vi "Average.vi"() -> ()   [LabVIEW 2011, in "Diamond Universal Driver.lvlib"]
uses:
  Diamond Universal Driver.lvlib
  Controls/dscBool.ctl
  Controls/board type.ctl
  Controls/dsccb.ctl
  constants.vi
  Controls/gain.ctl
  Controls/dscADSettings.ctl
  Controls/dscADScan.ctl
  support/dlls/mm32at.dll
  Controls/dscAIOint.ctl
  IO/DSCS.ctl
panel:
  out "status":T1 {"analog" items=["FALSE", "TRUE"]}
  out "aioint":T3 {"ch_align" items=["FALSE", "TRUE"]; "fifo en" items=["FALSE", "TRUE"]; "int clk gate" items=["FALSE", "TRUE"]; "ext gate en" items=["FALSE", "TRUE"]; "intclk" items=["FALSE", "TRUE"]; "cycle" items=["FALSE", "TRUE"]}
  out "ctVal":i32
  out "error out 2":errorcluster
  out "error":u8
  out "current time":timestamp
  out "sample_val":dbl[](array[numeric])
  out "error out":errorcluster
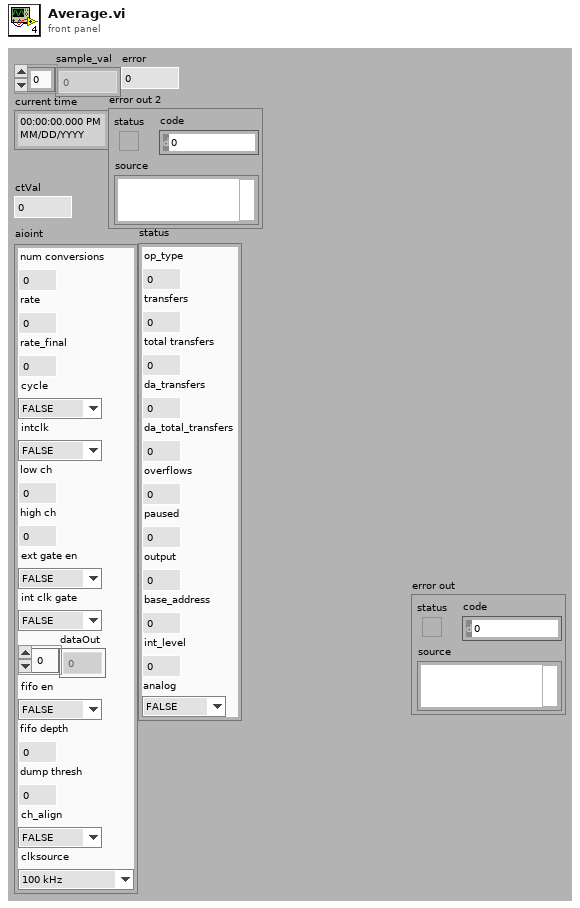
[diagram p1: front panel]
types:
  T1 = typedef "Diamond Universal Driver.lvlib/DSCS.ctl" = cluster{"op_type":u8, "transfers":u32, "total transfers":u32, "da_transfers":u32, "da_total_transfers":u32, "overflows":u32, "paused":u8, "output":u8, "base_address":u16, "int_level":u8, "analog":T2}
  T2 = typedef "dscBool.ctl" = i32
  T3 = typedef "Diamond Universal Driver.lvlib/dscAIOint.ctl" = cluster{"num conversions":u32, "rate":sgl, "rate_final":sgl, "cycle":T2, "intclk":T2, "low ch":u8, "high ch":u8, "ext gate en":T2, "int clk gate":T2, "dataOut":i16[], "fifo en":T2, "fifo depth":u16, "dump thresh":u32, "ch_align":T2, "clksource":enum8{"100 kHz", "1 MHz"}}
  T4 = typedef "dscADSettings.ctl" = cluster{"current_ch":u8, "gain":T5, "range":enum8{"RANGE_5", "RANGE_10"}, "polarity":enum16{"BIPOLAR", "UNIPOLAR"}, "load cal":u8, "scan_int":enum8{"20", "15", "10", "5", "9", "4"}, "addiff":enum8{"Single Ended", "Differential"}}
  T5 = typedef "gain.ctl" = enum8{"GAIN_1", "GAIN_2", "GAIN_8"}
  T6 = typedef "board type.ctl" = u8
  T7 = typedef "dsccb.ctl" = cluster{"board type":T6, "board num":i16, "base addr":u16, "int level":u8, "RMM external trig":T2, "RMM external trig c3":T2, "EMM IOAdd":u16[], "EMM IOInterrupt":u16[], "clkfreq0":enum8{"10 MHz", "1 MHz"}, "clkfreq1":enum8{"10 MHz", "1 MHz"}, "clksel1":enum8{"Internal (clkfrq1)", "External"}, "address space":dbl, "DAC cfg":u8, "clck_freq":i32, "dma_level":u8, "int_lvl 1":u8, "int_lvl 2":u8, "int_lvl 3":u8, "fpga":u16, "smm_ad_res":u8, "RMM mode 16bit":T2, "RMM DAC 0_3 ext en":T2, "RMM DAC 4_7 ext en":T2}
  T8 = typedef "dscADScan.ctl" = cluster{"low channel":u8, "high channel":u8, "sample_val":u16[], "gain":T5}
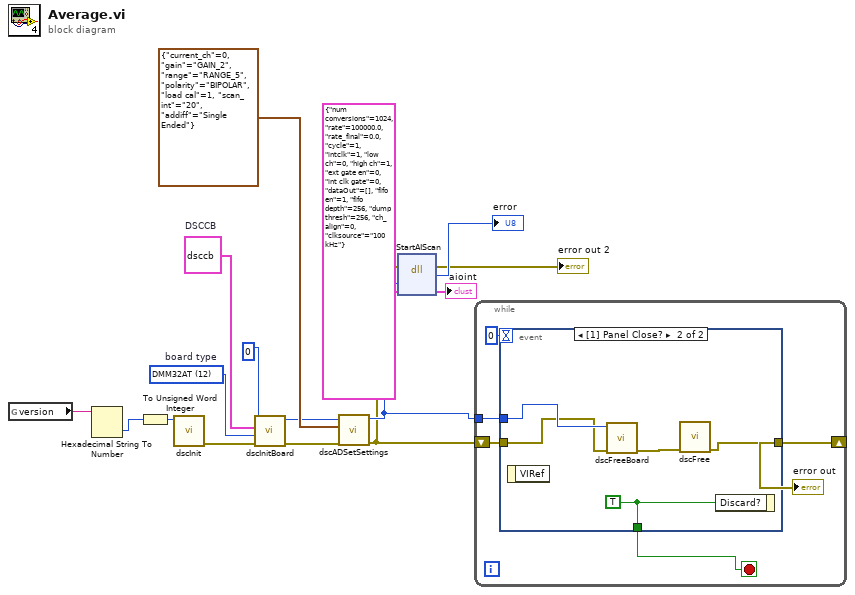
[diagram p0: block diagram]
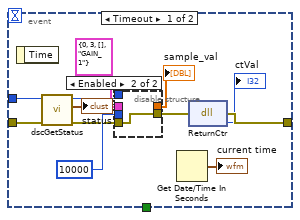
[diagram p2: hidden frame]
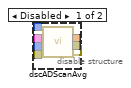
[diagram p3: hidden frame]
diagram:
  w12 = T6 12 items=["DMM16"=0, "RMM"=1, "TMM"=2, "OPMM"=3, "DMM"=4, "SMM"=5, "GMM"=6, "QMM"=7, "ZMM"=8, "PMM"=9, "OMM"=10, "RMM416"=11, "DMM32AT"=12, "EMMDIO"=13, "RMM1612"=14, "DMMAT"=15, "DMM16AT"=16, "IR104"=17, "EMM8"=18, "PROM"=19, "HERCEBX"=20, "CPT"=21, "DMM48AT"=22, "OMMIO"=23, "DIO82C55"=24, "ATHENA"=25, "METIS"=26, "DMM32XAT"=27, "ELEKTRA"=28, "GPIO11_9513"=29, "GPIO11_DIO"=30, "GPIO21"=31, "PSD"=32, "ATHENAII"=33, "DMM32DXAT"=34, "HELIOS"=35, "NEPTUNE"=36, "TEST"=126, "RAW"=127, "DRVR"=255]  # board type
  w10 = T7 {"board type"=12, "board num"=1, "base addr"=768, "int level"=3, "RMM external trig"=0, "RMM external trig c3"=0, "EMM IOAdd"=[0, 0, 0, 0, 0, 0, 0, 0], "EMM IOInterrupt"=[0, 0, 0, 0, 0, 0, 0, 0], "clkfreq0"=enum."10 MHz", "clkfreq1"=enum."10 MHz", "clksel1"=enum."Internal (clkfrq1)", "address space"=0.0, "DAC cfg"=0, "clck_freq"=0, "dma_level"=0, "int_lvl 1"=0, "int_lvl 2"=0, "int_lvl 3"=0, "fpga"=0, "smm_ad_res"=0, "RMM mode 16bit"=0, "RMM DAC 0_3 ext en"=0, "RMM DAC 4_7 ext en"=0}  # DSCCB
  n1 = global read "constants.vi" "version"() -> (w16:string)
  n2 = Hexadecimal String To Number(string=w16) -> (number=w14:u32)  [unwired: 2 in, 1 out]
  n3 = To Unsigned Word Integer(number=w14) -> (unsigned 16bit integer=w15:u16)
  n4 = call "dscInit.vi"("versionIn"=w15) -> ("error out"=w13:errorcluster)  [unwired: 9 in, 1 out]
  n5 = call "dscInitBoard.vi"("error in"=w13, "board type"=w12, "DSCCB"=w10, 11:u16 0 ("boardHandle")) -> ("error out"=w7:errorcluster, "boardHandleOut"=w8:i16)  [unwired: 5 in, 1 out]
  n6 = call "dscADSetSettings.vi"("error in"=w7, "adSettingsIn"=T4 {"current_ch"=0, "gain"=enum."GAIN_2", "range"=enum."RANGE_5", "polarity"=enum."BIPOLAR", "load cal"=1, "scan_int"=enum."20", "addiff"=enum."Single Ended"}, "boardIn"=w8) -> ("error out"=w4:errorcluster, "boardOut"=w5:i16)  [unwired: 6 in, 1 out]
  n7 = dll-call lib="C:/Users/mrichardson/Documents/Web Based Version Control SW/Reusable/Diamond Universal Driver/support/dlls/mm32at.dll" fn="StartAIScan"(error in=w4, "board"=w5, "aioint"=T3 {"num conversions"=1024, "rate"=100000.0, "rate_final"=0.0, "cycle"=1, "intclk"=1, "low ch"=0, "high ch"=1, "ext gate en"=0, "int clk gate"=0, "dataOut"=[], "fifo en"=1, "fifo depth"=256, "dump thresh"=256, "ch_align"=0, "clksource"=enum."100 kHz"} ("dscAIOint")) -> (error out=→"error out 2":errorcluster, "error"=→"error":u8, "aioint"=→"aioint":T3)  [unwired: 3 in, 1 out]
  n8 = while {
    tunnel: w5 -> [w19]
    shift-right: [w17] -> _
    shift-left: w4 -> [w18]
    stop <- w20 stop-if-true
    n9 = event shown="[1] Panel Close?" {
      selector: _ -> [_ _]
      dyn-events: _ -> [_ _]
      timeout: 0 -> [_ _]
      tunnel: [_ w45] -> w20
      tunnel: w19 -> [w26 w42]
      tunnel: w18 -> [w25 w41]
      tunnel: [w28 w43] -> w17
      event Timeout {
        n10 = event-data() -> ()  [unwired: 1 in, 1 out]
        n11 = call "dscGetStatus.vi"("error in"=w25, "board"=w26) -> ("error out"=w23:errorcluster, "status"=→"status":T1, "boardOut"=w24:i16)  [unwired: 7 in]
        n12 = disable-structure shown="Enabled" {
          disable-tunnel: [w39 _] -> w33
          disable-tunnel: 10000 ("count") -> [w38 _]
          disable-tunnel: T8 {"low channel"=0, "high channel"=3, "sample_val"=[], "gain"=enum."GAIN_1"} ("dscadscan") -> [w37 _]
          disable-tunnel: [w36 w40] -> w29
          disable-tunnel: w24 -> [w35 _]
          disable-tunnel: w23 -> [w34 w40]
          frame Disabled {
            n13 = call "dscADScanAvg.vi"("error in"=w34, "count"=w38, "dscadscan"=w37, "board"=w35) -> ("error out"=w36:errorcluster, "DataOut"=w39:cluster{"time":timestamp, "sample_val":sgl[]})  [unwired: 5 in, 1 out]
          }
          frame Enabled {
          }
        }
        "sample_val" <- w33
        n14 = Get Date/Time In Seconds() -> (seconds since 1Jan1904=→"current time":timestamp)
        n15 = dll-call lib="C:/Users/mrichardson/Documents/Web Based Version Control SW/Reusable/Diamond Universal Driver/support/dlls/mm32at.dll" fn="ReturnCtr"(error in=w29) -> (error out=w28:errorcluster, "ctVal"=→"ctVal":i32)  [unwired: 2 in, 1 out]
      }
      event Panel Close? {
        w45 = TRUE ("Discard?")
        n16 = event-data() -> ()  [unwired: 1 in, 1 out]
        n17 = call "dscFreeBoard.vi"("error in"=w41, "boardIn"=w42) -> ("error out"=w44:errorcluster)  [unwired: 8 in, 1 out]
        n18 = call "dscFree.vi"("error in"=w44) -> ("error out"=w43:errorcluster)  [unwired: 10 in]
        n19 = event-data("Discard?"=w45) -> ()  [unwired: 1 in, 1 out]
      }
    }
    "error out" <- w17
  }
